vi "CAM_pp3g_display.vi"(8 "Camera":T1="cam0", 9 "Log File Directory":refnum<vi>, 10 "Loop state Refnum":refnum<vi>, 11 "Image Ctl Refnum":refnum<vi>) -> ()   [LabVIEW 2013]
doc: "This VI is a general VI that loops through webcam images, and saves when necessary. It should be run asynchronously, so that webcam display/logging is independent of the main loop. Terminate this VI by setting the \"Webcam on\" value within the state info refnum to False."
uses:
  CTL_pp3g_LoopState.ctl
  pp3_CTL_BehavioralState.ctl
  CTL_pp3g_Trial.ctl
  pp3_CTL_TrialType.ctl
  labolabo2/waveforms/WFTypes.ctl
  <vilib>/userdefined/High Color/IMAQdx.ctl
  <vilib>/vision/Image Controls.llb/IMAQ Image.ctl
  <vilib>/vision/driver/NI_Vision_Acquisition_Software.lvlib
panel:
  out "error out":errorcluster
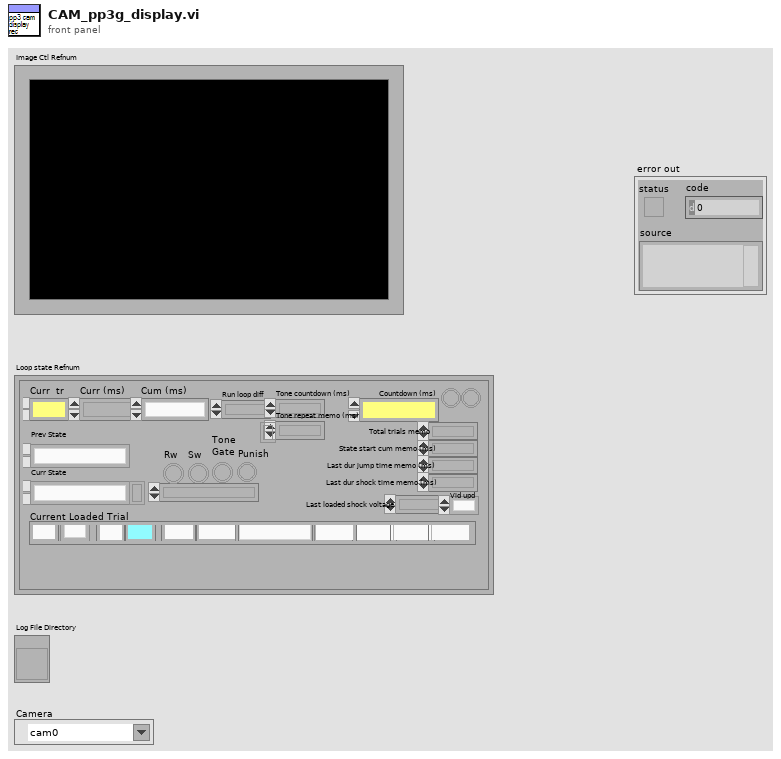
[diagram p1: front panel]
types:
  T1 = typedef "IMAQdx.ctl" = refnum<k21>
  T2 = typedef "CTL_pp3g_LoopState.ctl" = cluster{"Curr  tr":u16, "Curr (ms)":u32, "Cum (ms)":u64, "Run loop diff":i64, "Tone countdown (ms)":i64, "Countdown (ms)":i64, "Curr State":T3, "Prev State":T3, "Rw":bool, "Sw":bool, "Tone\nGate":bool, "Punish":bool, "Current DAQ DO Int":u16, "Current Loaded Trial":T4, "Total trials memo":i64, "State start cum memo (ms)":i64, "Last dur jump time memo (ms)":i64, "Last dur shock time memo (ms)":i64, "Tone repeat memo (ms)":i64, "Webcam on":bool, "Webcam recording":bool, "State update flag":bool, "Last loaded shock voltage":dbl, "Vid upd":enum16{"0", "1", "2", "3", "4", "5", "6", "7", "8", "9"}, "First time tone":bool}
  T3 = typedef "pp3_CTL_BehavioralState.ctl" = enum8{"0 NULL", "1 Habituation", "2 (Load Trial)", "3 Stay Period", "4 Load Audio/Click Delay", "5 GO Trial", "6 GO Jumped", "7 GO Timeout", "8 NOGO Trial", "9 NOGO Jumped", "10 NOGO Timeout", "11 TEST Trial", "12 TEST Jumped", "13 TEST Timeout", "14 Intertrial Interval", "15 Done"}
  T4 = typedef "CTL_pp3g_Trial.ctl" = cluster{"Trial Type Number":i16, "Trial Type":T5, "Trial Weight":u32, "Shock (mA)":dbl, "Duration (ms)":dbl, "Sound Type":T6, "Stim P1":dbl, "Stim P2":dbl, "Stim P3":dbl, "Stim P4":dbl, "DAQ Amplitude (V)":dbl}
  T5 = typedef "pp3_CTL_TrialType.ctl" = enum16{"OFF", "GO", "NOGO", "TEST"}
  T6 = typedef "WFTypes.ctl" = enum16{"00 NULL", "01 DC", "02 Noise", "03 Pure Tone", "04 FM Sweep", "05 FM Sweep BURST"}
  T7 = typedef "IMAQ Image.ctl" = refnum<image>
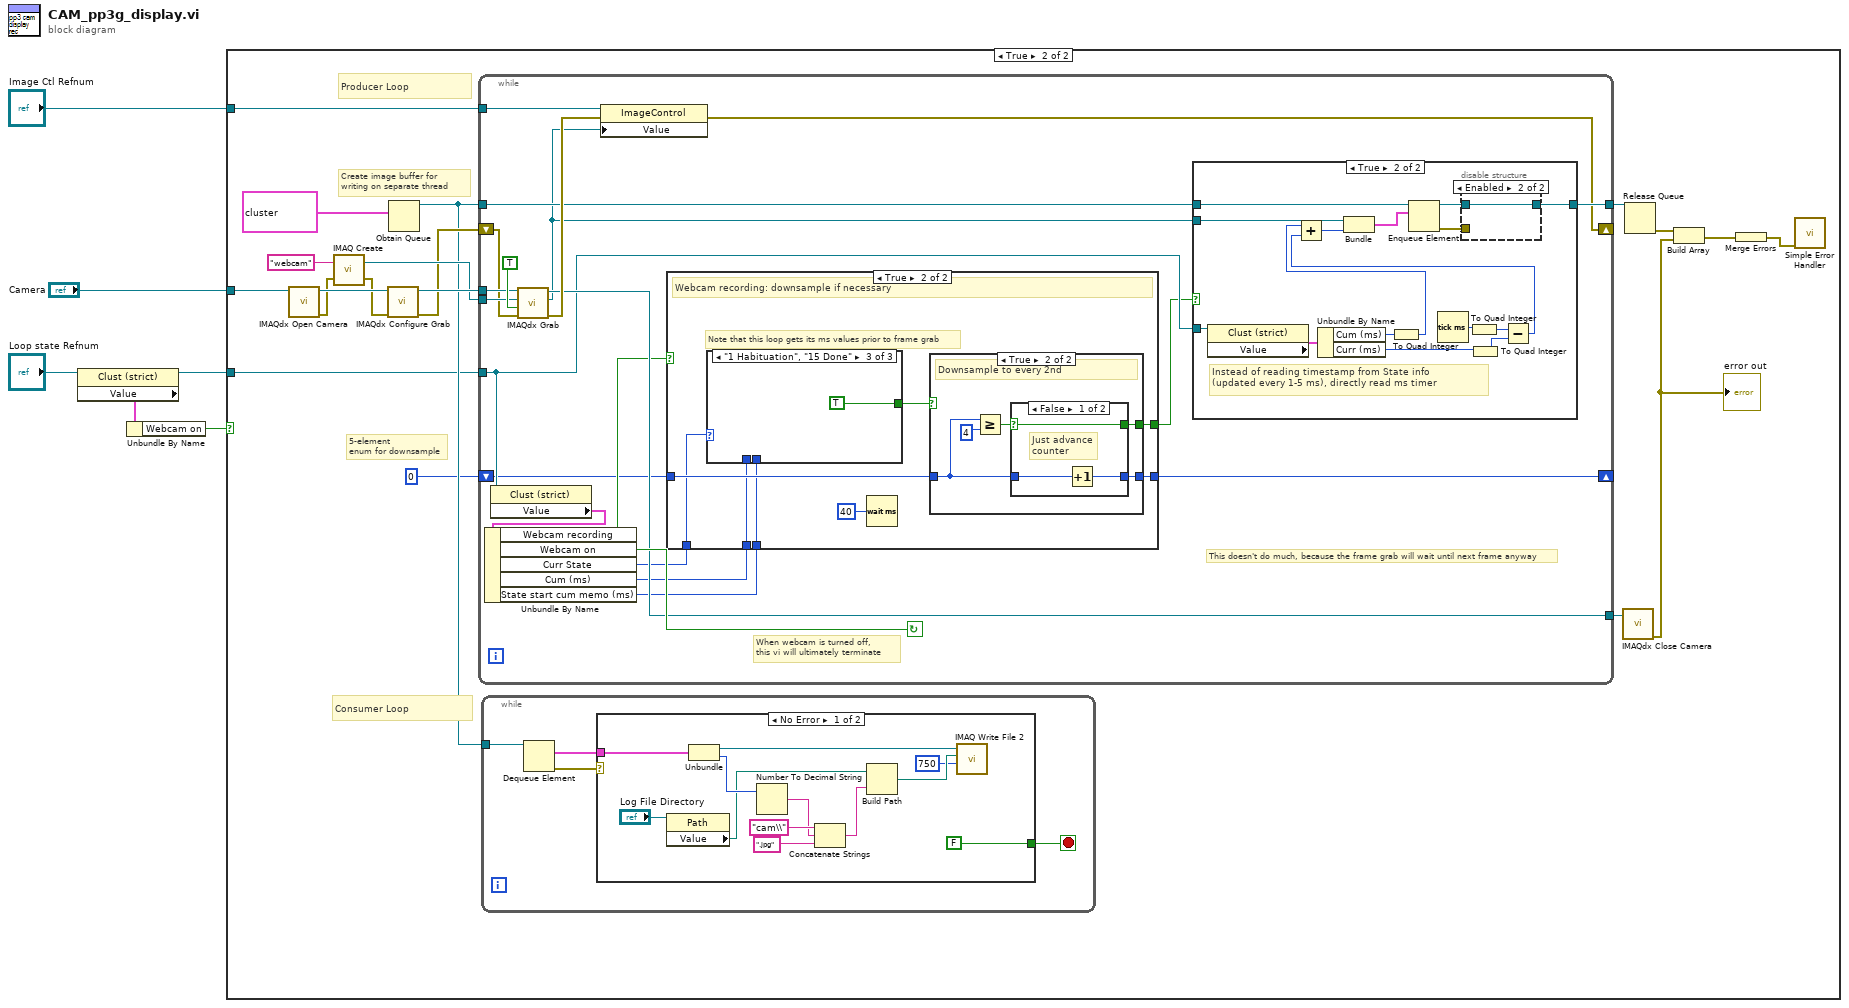
[diagram p0: block diagram]
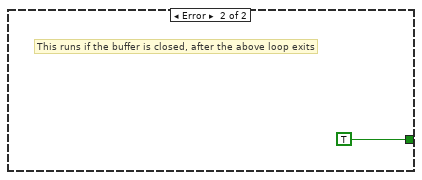
[diagram p3: hidden frame]
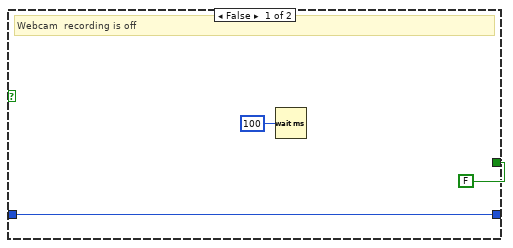
[diagram p4: hidden frame]
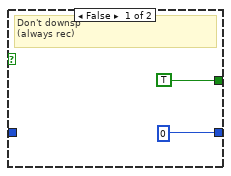
[diagram p5: hidden frame]
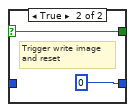
[diagram p6: hidden frame]
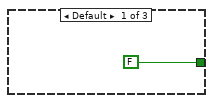
[diagram p7: hidden frame]
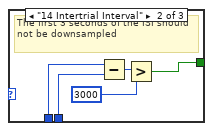
[diagram p8: hidden frame]
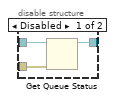
[diagram p10: hidden frame]
diagram:
  n1 = property class="Clust (strict)"(reference="Loop state Refnum") -> (reference out=w3:refnum<vi>, "Value"=w2:T2)  [unwired: 1 in, 1 out]
  n2 = Unbundle By Name(w2) -> ("Webcam on"=w1:bool)
  n3 = case shown="True" w1 {
    tunnel: "Image Ctl Refnum" -> [_ w25]
    tunnel: "Camera" -> [_ w21]
    tunnel: w3 -> [_ w8]
    frame False {
    }
    frame True {
      # "Consumer Loop"
      # "Producer Loop"
      # "5-element\nenum for downsample"
      # "Create image buffer for\nwriting on separate thread"
      n4 = call <vilib>:"IMAQdx Open Camera.vi"("Session In"=w21) -> ("error out"=w20:errorcluster, "Session Out"=w23:T1)  [unwired: 9 in]
      n5 = call "IMAQ Create"("Image Name"="webcam", "error in (no error)"=w20) -> ("New Image"=w17:T7, "error out"=w19:errorcluster)  [unwired: 3 in]
      n6 = call <vilib>:"IMAQdx Configure Grab.vi"("error in"=w19, "Session In"=w23) -> ("error out"=w11:errorcluster, "Session Out"=w18:T1)  [unwired: 8 in]
      n7 = Obtain Queue(element data type=cluster{"Image":T7, "Cum (ms)":i64} {"Image"="Webcam", "Cum (ms)"=0}) -> (queue out=w9:refnum<queue>)  [unwired: 4 in, 2 out]
      n8 = while {
        tunnel: w18 -> [w60]
        tunnel: w17 -> [w59]
        tunnel: w9 -> [w58]
        tunnel: [w56] -> w16
        tunnel: [w55] -> w12
        shift-right: [w52] -> _
        shift-left: w11 -> [w54]
        tunnel: w8 -> [w51]
        tunnel: w25 -> [w62]
        shift-right: [w46] -> _
        shift-left: 0 -> [w48]
        stop <- w57 continue-if-true
        # "This doesn't do much, because the frame grab will wait until next frame anyway"
        # "When webcam is turned off,\nthis vi will ultimately terminate"
        n9 = property class="Clust (strict)"(reference=w51) -> ("Value"=w49:T2)  [unwired: 1 in, 2 out]
        n10 = Unbundle By Name(w49) -> ("Webcam recording"=w50:bool, "Webcam on"=w57:bool, "Curr State"=w45:T3, "Cum (ms)"=w44:u64, "State start cum memo (ms)"=w43:i64)
        n11 = call <vilib>:"IMAQdx Grab.vi"("error in"=w54, "Wait for Next Buffer? (Yes)"=TRUE, "Image In"=w59, "Session In"=w60) -> ("error out"=w63:errorcluster, "Image Out"=w53:T7, "Session Out"=w56:T1)  [unwired: 4 in, 1 out]
        n12 = property class="ImageControl"(reference=w62, error in=w63, "Value"=w53) -> (error out=w52:errorcluster)  [unwired: 1 out]
        n13 = case shown="True" w50 {
          tunnel: w48 -> [w65 w71]
          tunnel: [FALSE w73] -> w47
          tunnel: [w65 w72] -> w46
          tunnel: w45 -> [_ w70]
          tunnel: w44 -> [_ w69]
          tunnel: w43 -> [_ w68]
          frame False {
            # "Webcam  recording is off"
            n14 = Wait (ms)(milliseconds to wait=u32 100) -> ()  [unwired: 1 out]
          }
          frame True {
            # "Note that this loop gets its ms values prior to frame grab"
            # "Webcam recording: downsample if necessary"
            n15 = case shown="\"1 Habituation\", \"15 Done\"" w70 {
              tunnel: [FALSE w90 TRUE] -> w74
              tunnel: w69 -> [_ w89 _]
              tunnel: w68 -> [_ w88 _]
              frame Default {
              }
              frame "14 Intertrial Interval" {
                # "The first 3 seconds of the ISI should not be downsampled"
                n16 = Subtract(x=w89, y=w88) -> (x-y=w92:u64)
                n17 = Greater?(x=w92, y=i64 3000) -> (0:w90:bool)
              }
              frame "1 Habituation", "15 Done" {
              }
            }
            n18 = Wait (ms)(milliseconds to wait=u32 40) -> ()  [unwired: 1 out]
            n19 = case shown="True" w74 {
              tunnel: [TRUE w77] -> w73
              tunnel: [0 w79] -> w72
              tunnel: w71 -> [_ w78]
              frame False {
                # "Don't downsp\n(always rec)"
              }
              frame True {
                # "Downsample to every 2nd"
                n20 = Greater Or Equal?(x=w78, y=4) -> (x >= y?=w80:bool)
                n21 = case shown="False" w80 {
                  selector: w80 -> [w82 w86]
                  tunnel: [w84 0] -> w79
                  tunnel: w78 -> [w83 _]
                  tunnel: [w82 w86] -> w77
                  frame False {
                    # "Just advance\ncounter"
                    n22 = Increment(x=w83) -> (x+1=w84:i32)
                  }
                  frame True {
                    # "Trigger write image\nand reset"
                  }
                }
              }
            }
          }
        }
        n23 = case shown="True" w47 {
          tunnel: w53 -> [_ w110]
          tunnel: w58 -> [w94 w109]
          tunnel: [w94 w107] -> w55
          tunnel: w51 -> [_ w105]
          frame False {
          }
          frame True {
            # "Instead of reading timestamp from State info\n(updated every 1-5 ms), directly read ms timer"
            n24 = property class="Clust (strict)"(reference=w105) -> ("Value"=w104:T2)  [unwired: 1 in, 2 out]
            n25 = Unbundle By Name(w104) -> ("Cum (ms)"=w96:u64, "Curr (ms)"=w100:u32)
            n26 = To Quad Integer(1:w96) -> (0:w95:i64)
            n27 = Tick Count (ms)() -> (millisecond timer value=w98:u32)
            n28 = To Quad Integer(1:w98) -> (0:w97:i64)
            n29 = To Quad Integer(1:w100) -> (0:w99:i64)
            n30 = Subtract(x=w97, y=w99) -> (x-y=w101:i64)
            n31 = Add(x=w95, y=w101) -> (x+y=w102:i64)
            n32 = Bundle("Image Out"=w110, w102) -> (w103:cluster{"Image Out":T7, i64})  [unwired: 1 in]
            n33 = Enqueue Element(queue=w109, element=w103) -> (queue out=w108:refnum<queue>, error out=w106:errorcluster)  [unwired: 2 in, 1 out]
            n34 = disable-structure shown="Enabled" {
              disable-tunnel: w108 -> [w113 w114]
              disable-tunnel: [w112 w114] -> w107
              disable-tunnel: w106 -> [w111 _]
              frame Disabled {
                n35 = Get Queue Status(queue=w113, error in (no error)=w111) -> (queue out=w112:refnum<queue>)  [unwired: 1 in, 7 out]
              }
              frame Enabled {
              }
            }
          }
        }
      }
      n36 = while {
        tunnel: w9 -> [w29]
        stop <- w27 stop-if-true
        n37 = Dequeue Element(queue=w29) -> (element=w26:cluster{"Image":T7, "Cum (ms)":i64}, error out=w28:errorcluster)  [unwired: 2 in, 2 out]
        n38 = case shown="No Error" w28 {
          tunnel: [FALSE TRUE] -> w27
          tunnel: w26 -> [w40 _]
          frame No Error {
            n39 = property class="Path"(reference="Log File Directory") -> ("Value"=w31:path)  [unwired: 1 in, 2 out]
            n40 = Unbundle(w40) -> ("Image"=w33:T7, "Cum (ms)"=w37:i64)
            n41 = Number To Decimal String(number=w37) -> (decimal integer string=w36:string)  [unwired: 1 in]
            n42 = Concatenate Strings("cam\\", w36, ".jpg" ("string")) -> (w35:string)
            n43 = Build Path(base path=w31, name or relative path=w35) -> (appended path=w34:path)
            n44 = call-poly "IMAQ Write File 2"("Image Quality"=u32 750, "File Path"=w34, "Image"=w33) -> ()  [unwired: 7 in, 2 out]
          }
          frame Error {
            # "This runs if the buffer is closed, after the above loop exits"
          }
        }
      }
      n45 = call <vilib>:"IMAQdx Close Camera.vi"("Session In"=w16) -> ("error out"=w10:errorcluster)  [unwired: 10 in]
      "error out" <- w10
      n46 = Release Queue(queue=w12) -> (error out=w15:errorcluster)  [unwired: 2 in, 2 out]
      n47 = Build Array(w15, w10) -> (w13:errorcluster[])
      n48 = Merge Errors(w13) -> (w14:errorcluster)
      n49 = call <vilib>:"Simple Error Handler.vi"("error in (no error)"=w14) -> ()  [unwired: 4 in, 5 out]
    }
  }
